vi "navX x_y_z (SubVI).vi"(0 "I2C Ref Out in":T1, 11 "error in (no error)":errorcluster) -> (4 "I2C Ref Out out":T1, 6 "value Z":ext, 8 "value Y":ext, 10 "value X":ext, 15 "error out":errorcluster)   [LabVIEW 2017]
uses:
  <vilib>/myRIO/Instrument Drivers/Onboard IO/I2C/typedefs/I2C Reference.ctl
  <vilib>/myRIO/Common/Instrument Driver Framework/Utilities/typedefs/myRIO Generic Hardware Reference.ctl
  <vilib>/myRIO/Common/Instrument Driver Framework/Utilities/typedefs/Hardware Version Enum.ctl
  <vilib>/myRIO/Common/Instrument Driver Framework/Utilities/typedefs/myRIO v1.0 Reference.ctl
  <vilib>/myRIO/Common/Instrument Driver Framework/Utilities/typedefs/Generic FPGA Reference.ctl
  <vilib>/myRIO/Common/Instrument Driver Framework/myRIO v1.0/I2C/typedefs/I2C Channels Enum.ctl
  <vilib>/myRIO/Instrument Drivers/Onboard IO/I2C/typedefs/I2C Configuration.ctl
  <vilib>/myRIO/Instrument Drivers/Onboard IO/I2C/typedefs/I2C Transfer Rate.ctl
  <vilib>/Utility/error.llb/Error Cluster From Error Code.vi
  <vilib>/myRIO/Common/Instrument Driver Framework/myRIO v1.0/I2C/vis/myRIO v1.0 Write I2C.vi
  <vilib>/myRIO/Common/Instrument Driver Framework/myRIO v1.0/I2C/vis/myRIO v1.0 Read I2C.vi
  <vilib>/myRIO/Instrument Drivers/Onboard IO/I2C/I2C.lvlib
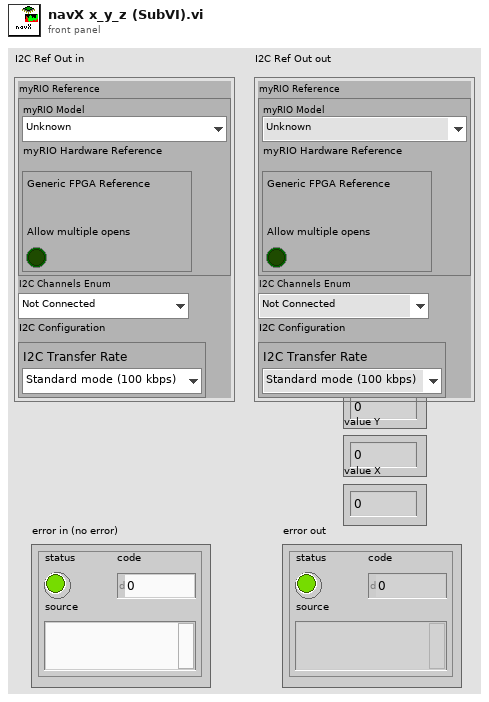
[diagram p1: front panel]
types:
  T1 = typedef "I2C.lvlib/I2C Reference.ctl" = cluster{"myRIO Reference":T2, "I2C Channels Enum":T6, "I2C Configuration":T7}
  T2 = typedef "myRIO Generic Hardware Reference.ctl" = cluster{"myRIO Model":T3, "myRIO Hardware Reference":T4}
  T3 = typedef "Hardware Version Enum.ctl" = enum16{"Unknown", "myRIO-1900", "myRIO-1950", "roboRIO", "NI ELVIS RIO CM"}
  T4 = typedef "myRIO v1.0 Reference.ctl" = cluster{"Generic FPGA Reference":T5, "Allow multiple opens":bool}
  T5 = typedef "Generic FPGA Reference.ctl" = refnum<k20>
  T6 = typedef "I2C Channels Enum.ctl" = enum16{"Not Connected", "A/I2C", "B/I2C", "I2C/I2C"}
  T7 = typedef "I2C.lvlib/I2C Configuration.ctl" = cluster{"I2C Transfer Rate":T8}
  T8 = typedef "I2C.lvlib/I2C Transfer Rate.ctl" = enum16{"Standard mode (100 kbps)", "Fast mode (400 kbps)"}
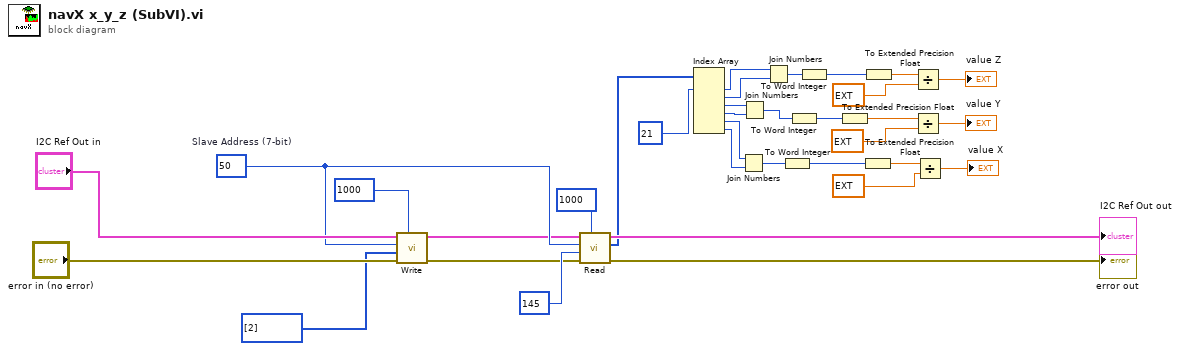
[diagram p0: block diagram]
diagram:
  w7 = u8 50  # Slave Address (7-bit)
  n1 = call <vilib>:"Write.vi"("Timeout ms (1000)"=1000, "error in (no error)"="error in (no error)", "Bytes to Write"=u8[] [2], "Slave Address (7-bit)"=w7, "I2C Ref In"="I2C Ref Out in") -> ("error out"=w1:errorcluster, "I2C Ref Out"=w3:T1)  [unwired: 5 in]
  n2 = call <vilib>:"Read.vi"("Timeout ms (1000)"=1000, "error in (no error)"=w1, "Byte Count"=u32 145, "Slave Address (7-bit)"=w7, "I2C Ref In"=w3) -> ("error out"=→"error out":errorcluster, "Bytes Read"=w8:u8[], "I2C Ref Out"=→"I2C Ref Out out":T1)  [unwired: 3 in]
  n3 = Index Array(array=w8, index #1=21 ("index")) -> (element #1=w13:u8, element #2=w10:u8, element #3=w15:u8, element #4=w16:u8, element #5=w18:u8, element #6=w19:u8)  [unwired: 5 in]
  n4 = Join Numbers(hi=w18, lo=w19) -> ((hi.lo)=w17:u16)
  n5 = Join Numbers(hi=w15, lo=w16) -> ((hi.lo)=w14:u16)
  n6 = Join Numbers(hi=w13, lo=w10) -> ((hi.lo)=w9:u16)
  n7 = To Word Integer(number=w17) -> (16bit integer=w21:i16)
  n8 = To Word Integer(number=w14) -> (16bit integer=w20:i16)
  n9 = To Word Integer(number=w9) -> (16bit integer=w11:i16)
  n10 = To Extended Precision Float(1:w20) -> (0:w25:ext)
  n11 = To Extended Precision Float(1:w21) -> (0:w27:ext)
  n12 = To Extended Precision Float(1:w11) -> (0:w26:ext)
  n13 = Divide(x=w26, y=ext 100.0) -> (x/y=→"value Z":ext)
  n14 = Divide(x=w25, y=ext 100.0) -> (x/y=→"value Y":ext)
  n15 = Divide(x=w27, y=ext 100.0) -> (x/y=→"value X":ext)
